vi "main_init_element_specs.vi"(6 "Simulation":refnum<vi>, 10 "Methane":refnum<vi>, 11 "Hydrolyse":refnum<vi>) -> ()   [LabVIEW 2019]
uses:
  lib/libSimulationControl/libSimulationControl.lvlib
panel:
  # "*******************************************************************\nBiogas Plant Control\n\nAuthor: Paul Zügel\nGCSC-Frankfurt am Main 2020\n\n*******************************************************************"
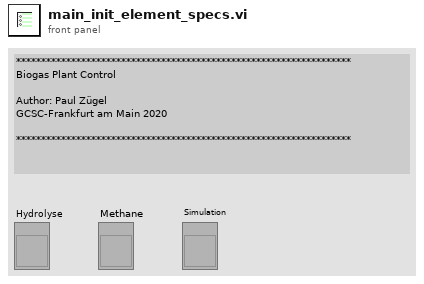
[diagram p1: front panel]
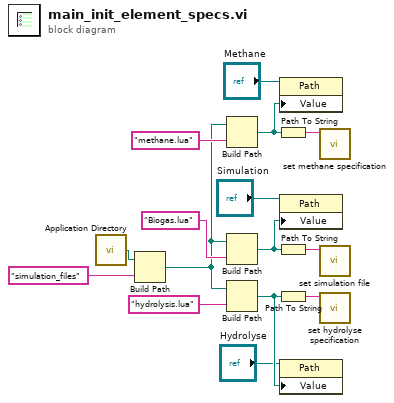
[diagram p0: block diagram]
diagram:
  n1 = call <vilib>:"Application Directory.vi"() -> ("Application Directory"=w4:path)
  n2 = Build Path(base path=w4, name or relative path="simulation_files") -> (appended path=w6:path)
  n3 = Build Path(base path=w6, name or relative path="methane.lua") -> (appended path=w14:path)
  n4 = Build Path(base path=w6, name or relative path="Biogas.lua") -> (appended path=w10:path)
  n5 = Build Path(base path=w6, name or relative path="hydrolysis.lua") -> (appended path=w15:path)
  n6 = Path To String(path=w14) -> (string=w13:string)
  n7 = Path To String(path=w10) -> (string=w11:string)
  n8 = Path To String(path=w15) -> (string=w12:string)
  n9 = property on="Property Node" class="Path"(reference="Methane", "Value"=w14) -> ()  [unwired: 1 in, 2 out]
  n10 = property on="Property Node" class="Path"(reference="Simulation", "Value"=w10) -> ()  [unwired: 1 in, 2 out]
  n11 = property on="Property Node" class="Path"(reference="Hydrolyse", "Value"=w15) -> ()  [unwired: 1 in, 2 out]
  n12 = call "set methane specification.vi"("methane_spec_file"=w13) -> ()  [unwired: 10 in, 1 out]
  n13 = call "set simulation file.vi"("sim_file"=w11) -> ()  [unwired: 10 in, 1 out]
  n14 = call "set hydrolyse specification.vi"("hydrolyse_spec_file"=w12) -> ()  [unwired: 10 in, 1 out]
